vi "Magnetic_FIeld.vi"(8 "error in (no error)":errorcluster, 9 "Choose Coil":string(combo)="Z", 10 "SMU":refnum<visa-resource-name>="GPIB0::1::INSTR", 11 "Power Supply":refnum<visa-resource-name>="GPIB0::6::INSTR") -> (0 "error out":errorcluster, 1 "Z mean 0 (Offset)":dbl=-0.03234 format="%0.2f", 2 "Z std dev":dbl=0.9189515543225985 format="%0.2f", 3 "Z Sensitivity LSB/mT":dbl=10.532150776053216)   [LabVIEW 2020]
uses:
  2b22404f-1e9c-45a2-8856-1edbb0e8605b.vi
  dd87499e-3bf9-4423-87a0-6918f72a918e.vi
  6e7286d9-0de1-421a-9aa3-658a620d422d.vi
  <vilib>/Analysis/baseanly.llb/Mean (DBL).vi
  Drivers/keithley_2450/Keithley 2450/Keithley 2450.lvlib
  Drivers/agilent_e363x_series/Agilent E363X Series/Agilent E363X Series.lvlib
  <vilib>/Analysis/NI_AALBase.lvlib
panel:
  out "Temp (C)":dbl=24.472 format="%0.2f"
  out "X std dev":dbl=0.16187463786473283 format="%0.2f"
  out "Y std dev":dbl=0.16944352892615727 format="%0.2f"
  out "X mean 0":dbl=0.26558 format="%0.2f"
  out "Y mean 0":dbl=0.18914 format="%0.2f"
  out "X mean NEG":dbl=1.3563200000000004 format="%0.2f"
  out "Y mean NEG":dbl=-0.38024000000000013 format="%0.2f"
  out "X mean POS mT":dbl=-0.9476600000000002 format="%0.2f"
  out "Y mean POS mT":dbl=0.8800400000000002 format="%0.2f"
  out "Z mean NEG":dbl=-9.317840000000002 format="%0.2f"
  out "Z mean POS mT":dbl=9.163979999999999 format="%0.2f"
  out "X ZERO":dbl=3.0
  out "Y ZERO":dbl=3.0
  out "X POS":dbl=-12.0
  out "Y POS":dbl=11.0
  out "X NEG":dbl=13.0
  out "Y NEG":dbl=-4.0
  out "Z NEG":dbl=-96.0
  out "Z ZERO":dbl
  out "Z POS":dbl=94.0
  out "noOfDevs out":u32=1
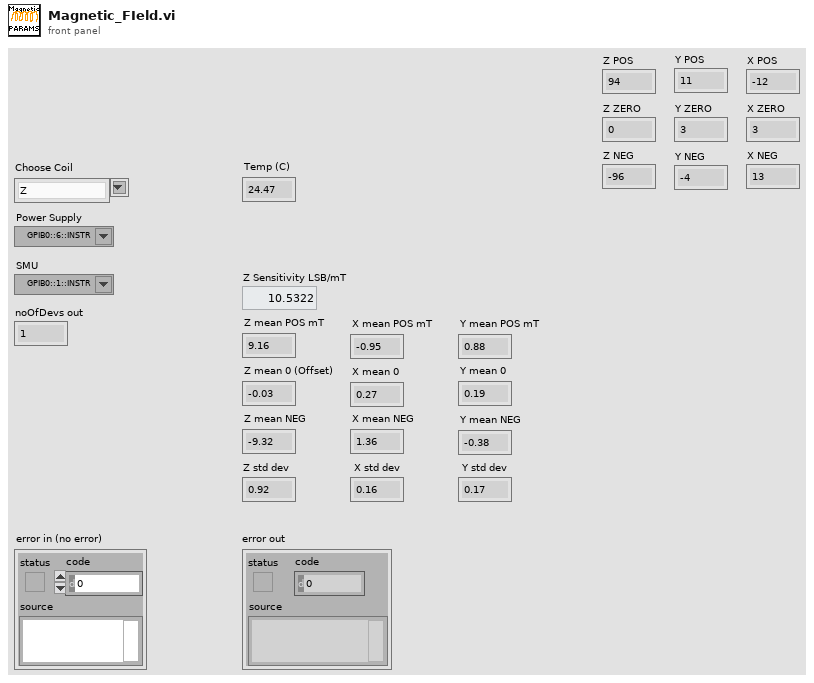
[diagram p1: front panel]
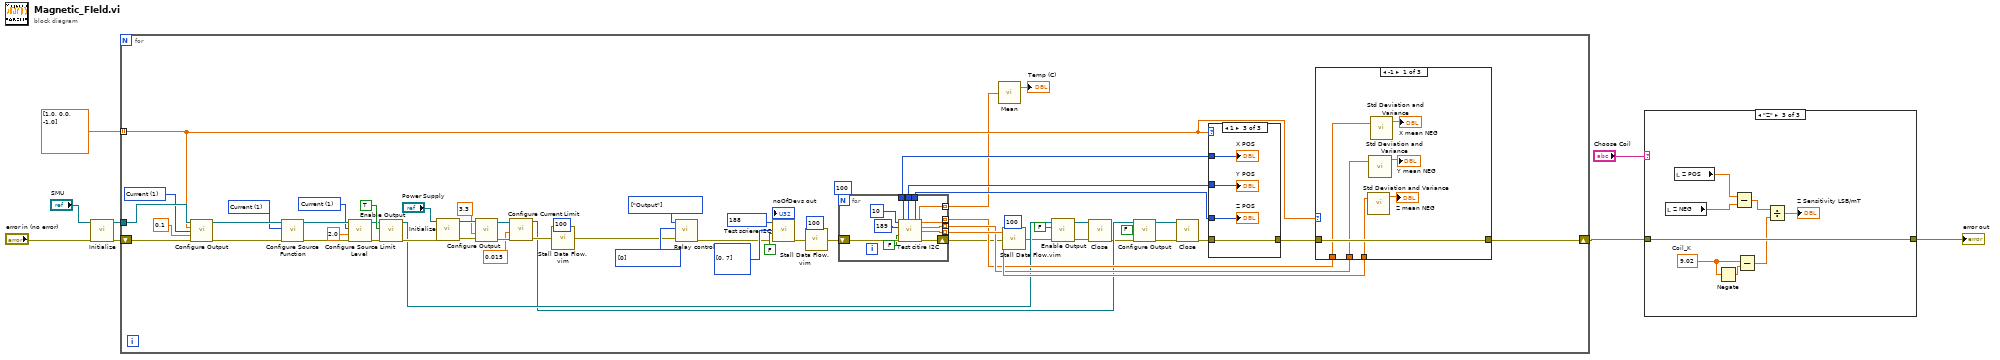
[diagram p0: block diagram]
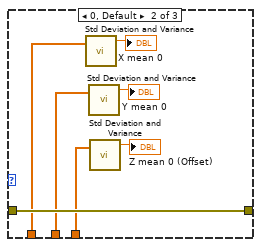
[diagram p4: hidden frame]
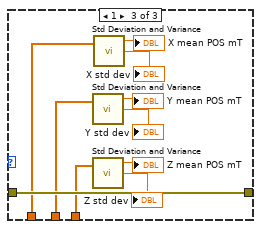
[diagram p5: hidden frame]
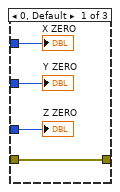
[diagram p6: hidden frame]
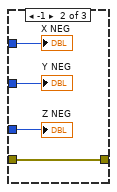
[diagram p7: hidden frame]
diagram:
  n1 = call "Initialize.vi"("error in (no error)"="error in (no error)", "VISA resource name"="SMU") -> ("error out"=w5:errorcluster, "VISA resource name out"=w6:refnum<visa-resource-name>)  [unwired: 8 in]
  n2 = for {
    tunnel: dbl[] [1.0, 0.0, -1.0] -> [w26] mode=indexing
    shift-right: [w27] -> w2
    shift-left: w5 -> [w66]
    tunnel: w6 -> [w67]
    w53 = u16[] [0] items=["low"=0, "high"=1, "Unchange"=255] ("outputValues")
    w54 = enum8{"Output", "Input", "Unchange"}[] [enum."Output"] items=["Output", "Input", "Unchange"] ("gpioDir")
    w56 = u16 1 items=["Volts", "Current"] ("Function (0: Volts)")
    w62 = u16 1 items=["Volts", "Current"] ("Function (0: Volts)")
    w63 = u16 1 items=["Voltage", "Current"] ("Source Mode  (0: Voltage)")
    n3 = call "Configure Output.vi"("VISA resource name"=w67, "Source Level (0)"=w26, "Source Mode  (0: Voltage)"=w63, "Source Limit Level (0.1)"=0.1, "error in (no error)"=w66) -> ("VISA resource name out"=w65:refnum<visa-resource-name>, "error out"=w64:errorcluster)  [unwired: 9 in]
    n4 = call "Configure Source Function.vi"("error in (no error)"=w64, "Function (0: Volts)"=w62, "VISA resource name"=w65) -> ("error out"=w60:errorcluster, "VISA resource name out"=w59:refnum<visa-resource-name>)  [unwired: 7 in]
    n5 = call "Configure Source Limit Level.vi"("error in (no error)"=w60, "Source Limit (1.0)"=2.0, "Function (0: Volts)"=w56, "VISA resource name"=w59) -> ("error out"=w57:errorcluster, "VISA resource name out"=w58:refnum<visa-resource-name>)  [unwired: 6 in]
    n6 = call "Enable Output.vi"("error in (no error)"=w57, "Enable Output (T: Enable)"=TRUE, "VISA resource name"=w58) -> ("error out"=w47:errorcluster, "VISA resource name out"=w22:refnum<visa-resource-name>)  [unwired: 7 in]
    n7 = call "Initialize.vi"("error in (no error)"=w47, "VISA resource name"="Power Supply") -> ("error out"=w46:errorcluster, "VISA resource name out"=w43:refnum<visa-resource-name>)  [unwired: 8 in]
    n8 = call "Configure Output.vi"("error in (no error)"=w46, "Voltage Level (0.0 V)"=3.3, "VISA resource name"=w43) -> ("error out"=w45:errorcluster, "VISA resource name out"=w41:refnum<visa-resource-name>)  [unwired: 7 in]
    n9 = call "Configure Current Limit.vi"("error in (no error)"=w45, "Current Limit (0.0 A)"=0.015, "VISA resource name"=w41) -> ("error out"=w39:errorcluster, "VISA resource name out"=w18:refnum<visa-resource-name>)  [unwired: 7 in]
    n10 = call "Stall Data Flow.vim"("value in"=w39, "milliseconds to wait"=u32 100) -> ("value out"=w38:errorcluster)  [unwired: 1 out]
    n11 = call "Relay control.vi"("error in (no error) 2"=w38, "outputValues"=w53, "gpioDir"=w54) -> ("error out"=w48:errorcluster)  [unwired: 8 in]
    n12 = call "Test scriere I2C.vi"("error in (no error)"=w48, "use7bitAddress"=FALSE, "i2cTxData"=u8[] [0, 7], "slaveAddress"=u8 188) -> ("error out"=w36:errorcluster, "noOfDevs out"=→"noOfDevs out":u32)  [unwired: 5 in, 1 out]
    n13 = call "Stall Data Flow.vim"("value in"=w36, "milliseconds to wait"=u32 100) -> ("value out"=w35:errorcluster)  [unwired: 1 out]
    n14 = for {
      N: 100 -> [_]
      tunnel: [w99] -> w23 mode=indexing
      tunnel: [w98] -> w24 mode=indexing
      tunnel: [w97] -> w25 mode=indexing
      shift-right: [w102] -> w13
      shift-left: w35 -> [w104]
      tunnel: [w96] -> w10 mode=indexing
      tunnel: [w95] -> w31
      tunnel: [w94] -> w30
      tunnel: [w93] -> w29
      n15 = call "Test citire I2C.vi"("bytesToRead"=u32 10, "slaveAddress"=u8 189, "use7bitAddress"=FALSE, "error in (no error)"=w104) -> ("12 bit LSB value (x)"=w93:i32, "12 bit LSB value (y)"=w94:i32, "12 bit LSB value (z)"=w95:i32, "12 bit Field value (mT) X"=w99:dbl, "12 bit Field value (mT) Y"=w98:dbl, "12 bit Field value (mT) Z"=w97:dbl, "12 bit temp (C)"=w96:dbl, "error out"=w102:errorcluster)  [unwired: 2 in, 2 out]
    }
    n16 = call-poly <vilib>:"Mean.vi"("X"=w10) -> ("mean"=→"Temp (C)":dbl)  [unwired: 1 out]
    n17 = call "Stall Data Flow.vim"("value in"=w13, "milliseconds to wait"=u32 100) -> ("value out"=w12:errorcluster)  [unwired: 1 out]
    n18 = call "Enable Output.vi"("error in (no error)"=w12, "Enable Output (T: Enable)"=FALSE, "VISA resource name"=w22) -> ("error out"=w20:errorcluster, "VISA resource name out"=w21:refnum<visa-resource-name>)  [unwired: 7 in]
    n19 = call "Close.vi"("error in (no error)"=w20, "VISA resource name"=w21) -> ("error out"=w16:errorcluster)  [unwired: 9 in]
    n20 = call "Configure Output.vi"("Enable Output (T: Enable)"=FALSE, "error in (no error)"=w16, "VISA resource name"=w18) -> ("error out"=w15:errorcluster, "VISA resource name out"=w17:refnum<visa-resource-name>)  [unwired: 7 in]
    n21 = call "Close.vi"("error in (no error)"=w15, "VISA resource name"=w17) -> ("error out"=w32:errorcluster)  [unwired: 9 in]
    n22 = case shown="1" w26 {
      tunnel: w32 -> [w107 w111 w116]
      tunnel: [w107 w111 w116] -> w28
      tunnel: w31 -> [w108 w112 w115]
      tunnel: w30 -> [w105 w109 w113]
      tunnel: w29 -> [w106 w110 w114]
      frame 0, Default {
        "Z ZERO" <- w108
        "Y ZERO" <- w105
        "X ZERO" <- w106
      }
      frame -1 {
        "Z NEG" <- w112
        "Y NEG" <- w109
        "X NEG" <- w110
      }
      frame 1 {
        "Z POS" <- w115
        "Y POS" <- w113
        "X POS" <- w114
      }
    }
    n23 = case shown="-1" w26 {
      tunnel: w28 -> [w75 w81 w92]
      tunnel: [w75 w81 w92] -> w27
      tunnel: w25 -> [w73 w80 w90]
      tunnel: w24 -> [w70 w77 w87]
      tunnel: w23 -> [w69 w76 w86]
      frame -1 {
        n24 = call <vilib>:"Std Deviation and Variance.vi"("X"=w73) -> ("mean"=→"Z mean NEG":dbl)  [unwired: 1 in, 2 out]
        n25 = call <vilib>:"Std Deviation and Variance.vi"("X"=w70) -> ("mean"=→"Y mean NEG":dbl)  [unwired: 1 in, 2 out]
        n26 = call <vilib>:"Std Deviation and Variance.vi"("X"=w69) -> ("mean"=→"X mean NEG":dbl)  [unwired: 1 in, 2 out]
      }
      frame 0, Default {
        n27 = call <vilib>:"Std Deviation and Variance.vi"("X"=w76) -> ("mean"=→"X mean 0":dbl)  [unwired: 1 in, 2 out]
        n28 = call <vilib>:"Std Deviation and Variance.vi"("X"=w77) -> ("mean"=→"Y mean 0":dbl)  [unwired: 1 in, 2 out]
        n29 = call <vilib>:"Std Deviation and Variance.vi"("X"=w80) -> ("mean"=→"Z mean 0 (Offset)":dbl)  [unwired: 1 in, 2 out]
      }
      frame 1 {
        n30 = call <vilib>:"Std Deviation and Variance.vi"("X"=w87) -> ("mean"=→"Y mean POS mT":dbl, "standard deviation"=→"Y std dev":dbl)  [unwired: 1 in, 1 out]
        n31 = call <vilib>:"Std Deviation and Variance.vi"("X"=w90) -> ("mean"=→"Z mean POS mT":dbl, "standard deviation"=→"Z std dev":dbl)  [unwired: 1 in, 1 out]
        n32 = call <vilib>:"Std Deviation and Variance.vi"("X"=w86) -> ("mean"=→"X mean POS mT":dbl, "standard deviation"=→"X std dev":dbl)  [unwired: 1 in, 1 out]
      }
    }
  }
  n33 = case shown="\"Z\"" "Choose Coil" {
    tunnel: [w117 w118 w126] -> w3
    tunnel: w2 -> [w117 w118 w126]
    frame "X", Default {
    }
    frame "Y" {
    }
    frame "Z" {
      w121 = 9.02  # Coil_K
      n34 = local read "Z NEG"() -> (w124:dbl)
      n35 = local read "Z POS"() -> (w125:dbl)
      n36 = Negate(x=w121) -> (-x=w120:dbl)
      n37 = Subtract(x=w125, y=w124) -> (x-y=w123:dbl)
      n38 = Subtract(x=w121, y=w120) -> (x-y=w119:dbl)
      n39 = Divide(x=w123, y=w119) -> (x/y=→"Z Sensitivity LSB/mT":dbl)
    }
  }
  "error out" <- w3
